vi "BI_VFFT plot 0.5.vi"() -> ()   [LabVIEW 2021]
uses:
  <vilib>/Utility/file.llb/Read Delimited Spreadsheet (DBL).vi
panel:
  out "IV":cluster{dbl[], "Intensity V vs I and B":dbl[]}(graph)
  out "Intensity V vs I and B":dbl[][](graph)
  out "Intensity FFT vs B with fix I":dbl[][](graph)
  out "FFT at fix B and I":cluster{dbl[], "Intensity V vs I and B":dbl[]}(graph)
  out "Intensity FFT vs I with fix B":dbl[][](graph)
  out "FFT at fix I and B":cluster{dbl[], "Intensity V vs I and B":dbl[]}(graph)
  out "I index":i32=30
  out "B index":i32=11
  out "parameter rows":dbl[][](array[numeric])
  out "data rows":dbl[][](array[numeric])
  out "field rows":dbl[][](array[numeric])
  out "Cursor I":dbl=0.29559164733178656
  out "Cursor B":dbl=-0.6575098814229249
  in  "Load":bool
  in  "Stop":bool
  in  "Book number":i32=685
  in  "parent data folder":path=path "C:/Users/gyue/Box/Guang Yue uiuc research box folder/data/Contour plot"
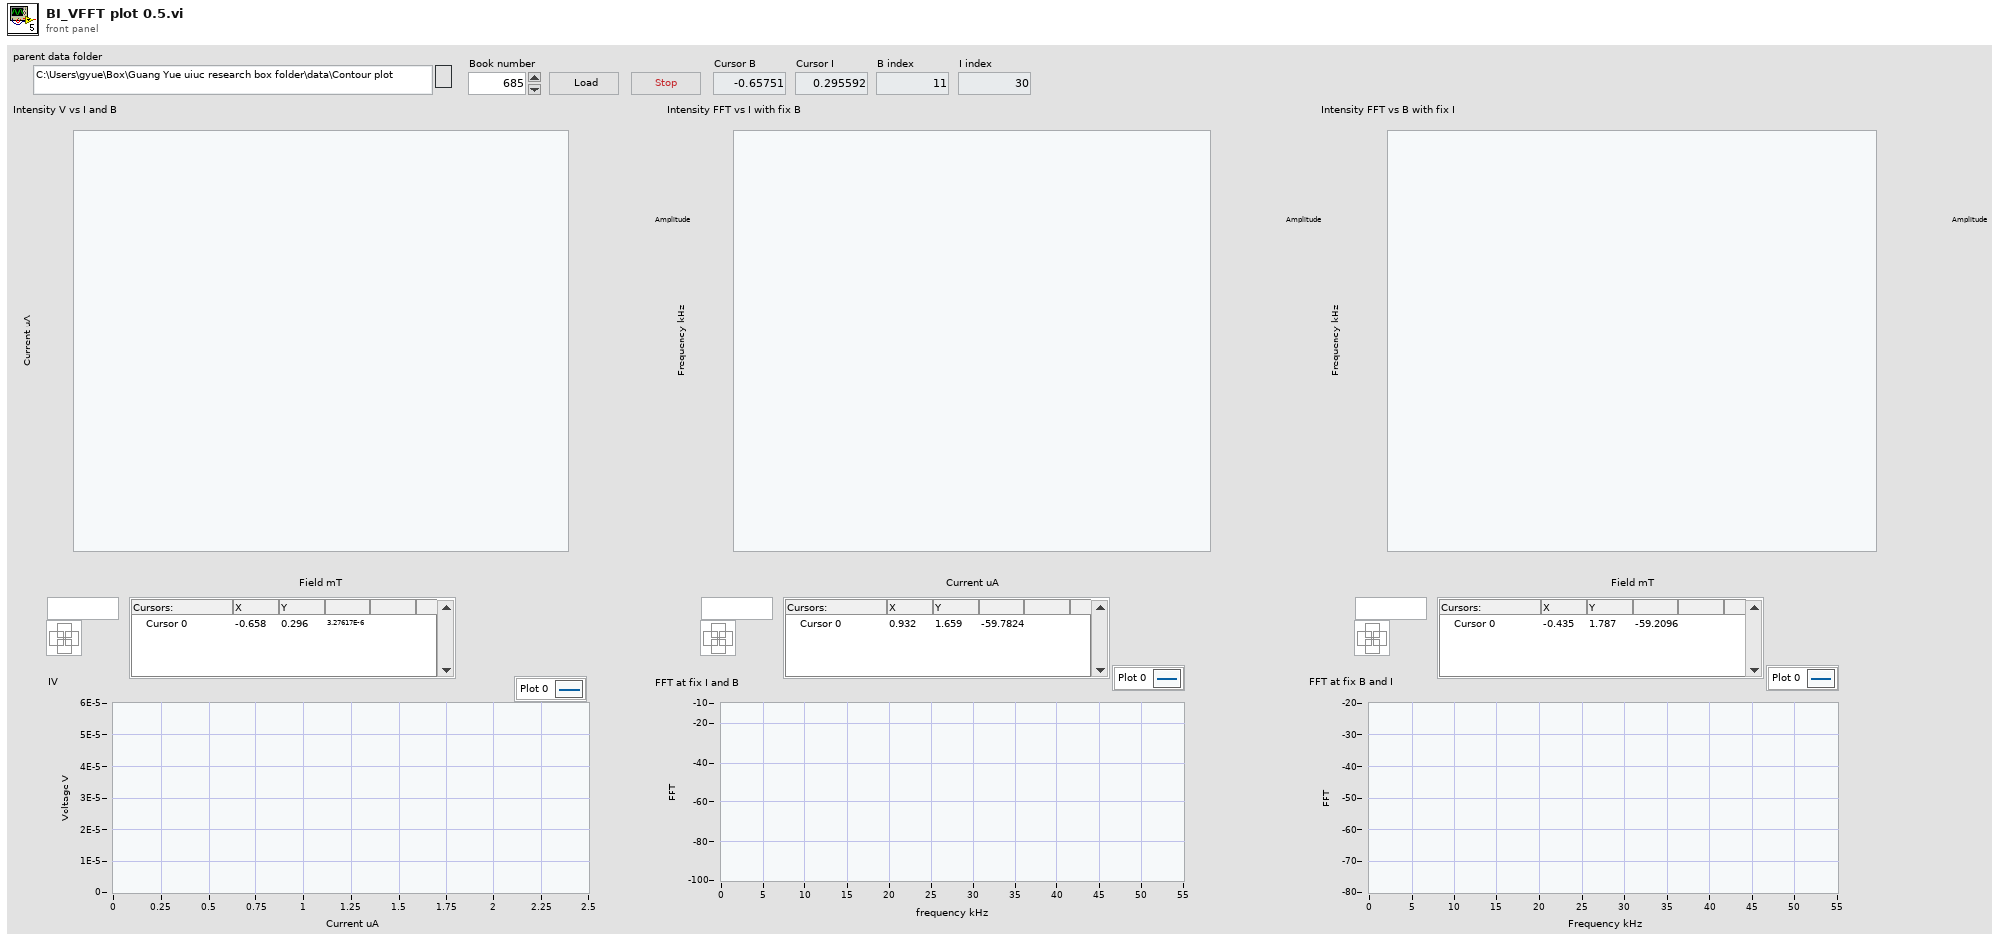
[diagram p1: front panel]
types:
  T1 = cluster{"B offset":dbl, "B multiply":dbl, "I offset":dbl, "I multiply":dbl}
  T2 = cluster{"x offset":dbl, "x multiply":dbl, "y offset":dbl, "y multiply":dbl}
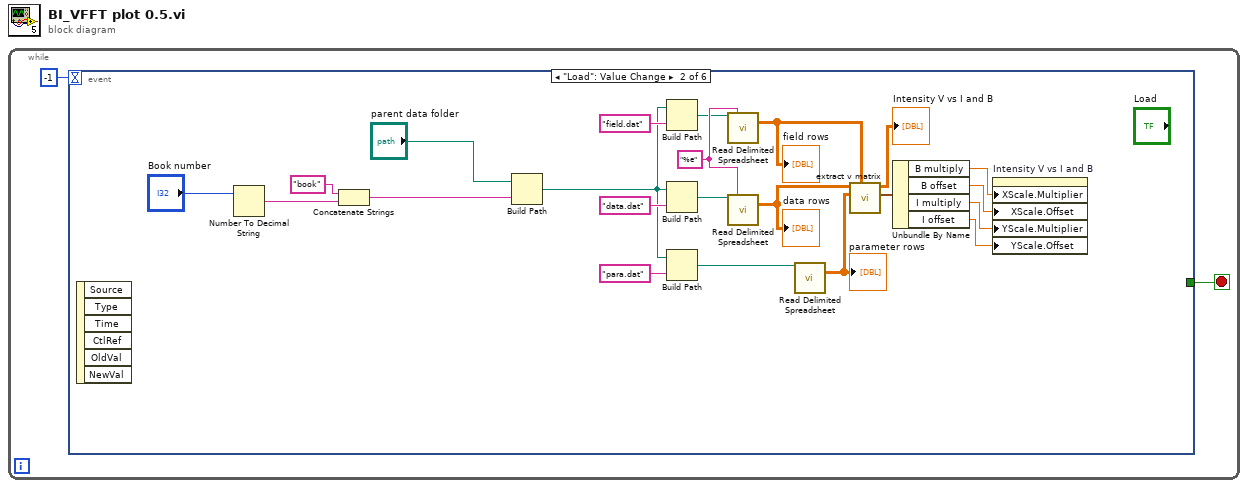
[diagram p0: block diagram]
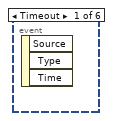
[diagram p2: hidden frame]
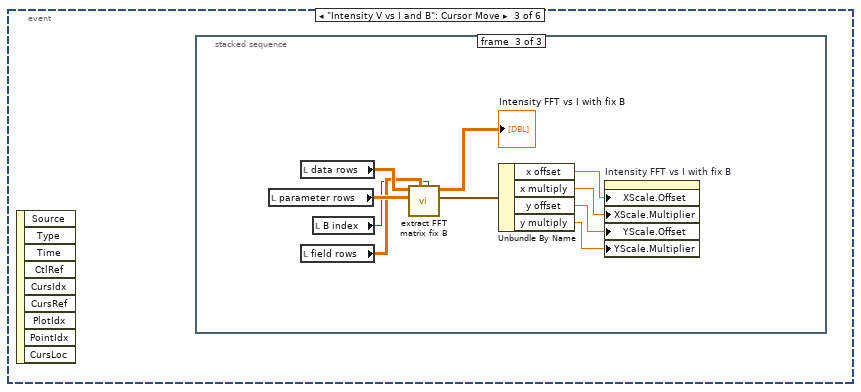
[diagram p3: hidden frame]
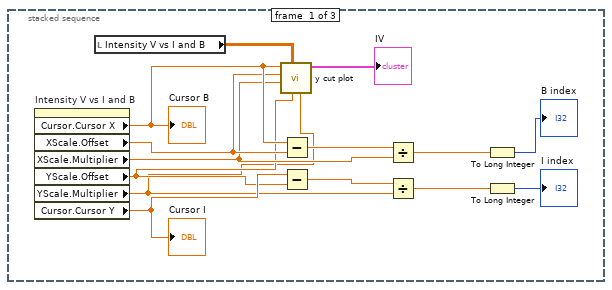
[diagram p4: hidden frame]
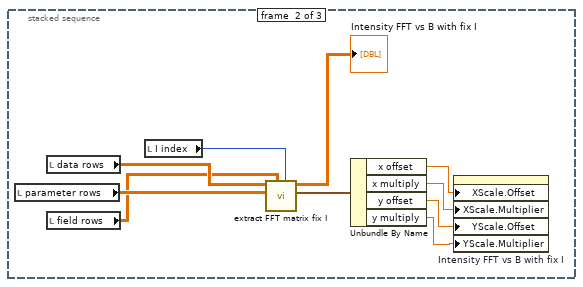
[diagram p5: hidden frame]
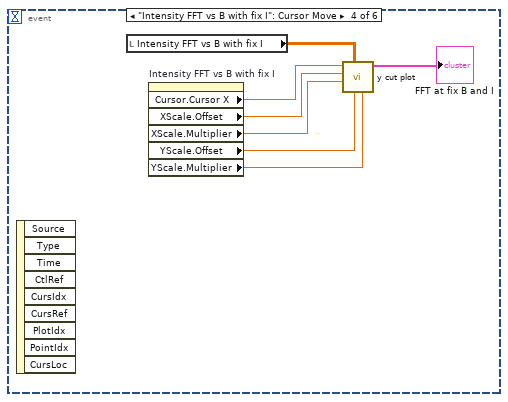
[diagram p6: hidden frame]
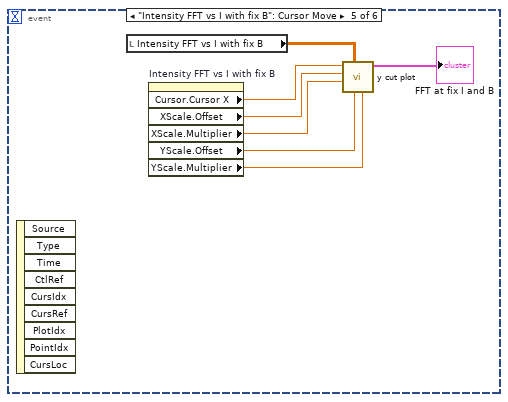
[diagram p7: hidden frame]
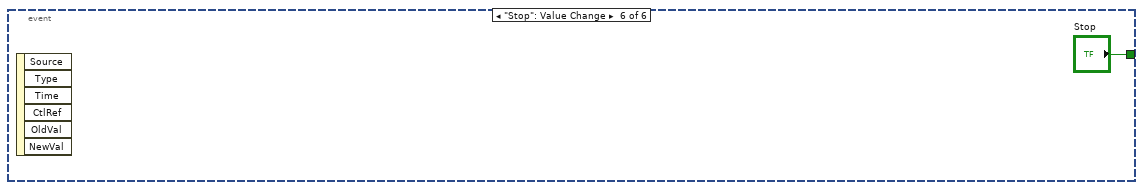
[diagram p8: hidden frame]
diagram:
  n1 = while {
    stop <- w1 stop-if-true
    n2 = event shown="[1] \"Load\": Value Change" {
      selector: _ -> [_ _ _ _ _ _]
      dyn-events: _ -> [_ _ _ _ _ _]
      timeout: -1 -> [_ _ _ _ _ _]
      tunnel: [_ _ _ _ _ "Stop"] -> w1
      event Timeout {
        n3 = event-data() -> ()  [unwired: 1 in, 3 out]
      }
      event "Load": Value Change {
        w15 = "%e" ("format (%.3f)")
        n4 = event-data() -> ()  [unwired: 1 in, 6 out]
        n5 = Number To Decimal String(number="Book number") -> (decimal integer string=w21:string)  [unwired: 1 in]
        n6 = Concatenate Strings("book" ("string"), w21) -> (w20:string)
        n7 = Build Path(base path="parent data folder", name or relative path=w20) -> (appended path=w16:path)
        n8 = Build Path(base path=w16, name or relative path="field.dat") -> (appended path=w13:path)
        n9 = Build Path(base path=w16, name or relative path="data.dat") -> (appended path=w14:path)
        n10 = Build Path(base path=w16, name or relative path="para.dat") -> (appended path=w12:path)
        n11 = call-poly <vilib>:"Read Delimited Spreadsheet.vi"("file path (dialog if empty)"=w13, "format (%.3f)"=w15) -> ("all rows"=w3:dbl[][])  [unwired: 8 in, 5 out]
        "field rows" <- w3
        n12 = call-poly <vilib>:"Read Delimited Spreadsheet.vi"("file path (dialog if empty)"=w14, "format (%.3f)"=w15) -> ("all rows"=w10:dbl[][])  [unwired: 8 in, 5 out]
        "data rows" <- w10
        n13 = call-poly <vilib>:"Read Delimited Spreadsheet.vi"("file path (dialog if empty)"=w12) -> ("all rows"=w11:dbl[][])  [unwired: 9 in, 5 out]
        "parameter rows" <- w11
        n14 = call "extract v matrix.vi"("all field rows"=w3, "parameter"=w11, "all data rows"=w10) -> ("plot parameter"=w8:T1, "V matrix"=→"Intensity V vs I and B":dbl[][])  [unwired: 7 in]
        n15 = Unbundle By Name(w8) -> ("B multiply"=w7:dbl, "B offset"=w6:dbl, "I multiply"=w5:dbl, "I offset"=w4:dbl)
        n16 = property on="Intensity V vs I and B" class="IntGraph (strict)"("XScale.Multiplier"=w7, "XScale.Offset"=w6, "YScale.Multiplier"=w5, "YScale.Offset"=w4) -> ()  [unwired: 2 in, 2 out]
      }
      event "Intensity V vs I and B": Cursor Move {
        n17 = event-data() -> ()  [unwired: 1 in, 9 out]
        n18 = stacked-sequence {
          frame #0 {
            n19 = property on="Intensity V vs I and B" class="IntGraph (strict)"() -> ("Cursor.Cursor X"=w36:dbl, "XScale.Offset"=w35:dbl, "XScale.Multiplier"=w33:dbl, "YScale.Offset"=w27:dbl, "YScale.Multiplier"=w26:dbl, "Cursor.Cursor Y"=w28:dbl)  [unwired: 2 in, 2 out]
            "Cursor B" <- w36
            "Cursor I" <- w28
            n20 = local read "Intensity V vs I and B"() -> (w38:dbl[][])
            n21 = call "y cut plot.vi"("YScale.Multiplier"=w26, "YScale.Offset"=w27, "Intensity V vs I and B"=w38, "XScale.Multiplier"=w33, "XScale.Offset"=w35, "Cursor.Cursor X"=w36) -> ("Cluster"=→"IV":cluster{dbl[], "Intensity V vs I and B":dbl[]})  [unwired: 5 in]
            n22 = Subtract(x=w36, y=w35) -> (x-y=w34:dbl)
            n23 = Subtract(x=w28, y=w27) -> (x-y=w30:dbl)
            n24 = Divide(x=w34, y=w33) -> (x/y=w32:dbl)
            n25 = Divide(x=w30, y=w26) -> (x/y=w29:dbl)
            n26 = To Long Integer(number=w32) -> (32bit integer=→"B index":i32)
            n27 = To Long Integer(number=w29) -> (32bit integer=→"I index":i32)
          }
          frame #1 {
            n28 = local read "parameter rows"() -> (w47:dbl[][])
            n29 = local read "data rows"() -> (w48:dbl[][])
            n30 = local read "field rows"() -> (w46:dbl[][])
            n31 = local read "I index"() -> (w44:i32)
            n32 = call "extract FFT matrix fix I.vi"("I index"=w44, "all field rows"=w46, "parameter"=w47, "all data rows"=w48) -> ("plot parameter"=w45:T2, "FFT matrix"=→"Intensity FFT vs B with fix I":dbl[][])  [unwired: 6 in]
            n33 = Unbundle By Name(w45) -> ("x offset"=w42:dbl, "x multiply"=w41:dbl, "y offset"=w40:dbl, "y multiply"=w39:dbl)
            n34 = property on="Intensity FFT vs B with fix I" class="IntGraph (strict)"("XScale.Offset"=w42, "XScale.Multiplier"=w41, "YScale.Offset"=w40, "YScale.Multiplier"=w39) -> ()  [unwired: 2 in, 2 out]
          }
          frame #2 {
            n35 = local read "parameter rows"() -> (w57:dbl[][])
            n36 = local read "data rows"() -> (w58:dbl[][])
            n37 = local read "field rows"() -> (w56:dbl[][])
            n38 = local read "B index"() -> (w55:i32)
            n39 = call "extract FFT matrix fix B.vi"("B index"=w55, "all field rows"=w56, "parameter"=w57, "all data rows"=w58) -> ("plot parameter"=w53:T2, "FFT matrix"=→"Intensity FFT vs I with fix B":dbl[][])  [unwired: 6 in]
            n40 = Unbundle By Name(w53) -> ("x offset"=w52:dbl, "x multiply"=w51:dbl, "y offset"=w50:dbl, "y multiply"=w49:dbl)
            n41 = property on="Intensity FFT vs I with fix B" class="IntGraph (strict)"("XScale.Offset"=w52, "XScale.Multiplier"=w51, "YScale.Offset"=w50, "YScale.Multiplier"=w49) -> ()  [unwired: 2 in, 2 out]
          }
        }
      }
      event "Intensity FFT vs B with fix I": Cursor Move {
        n42 = event-data() -> ()  [unwired: 1 in, 9 out]
        n43 = local read "Intensity FFT vs B with fix I"() -> (w65:dbl[][])
        n44 = property on="Intensity FFT vs B with fix I" class="IntGraph (strict)"() -> ("Cursor.Cursor X"=w64:dbl, "XScale.Offset"=w63:dbl, "XScale.Multiplier"=w62:dbl, "YScale.Offset"=w60:dbl, "YScale.Multiplier"=w59:dbl)  [unwired: 2 in, 2 out]
        n45 = call "y cut plot.vi"("YScale.Multiplier"=w59, "YScale.Offset"=w60, "Intensity V vs I and B"=w65, "XScale.Multiplier"=w62, "XScale.Offset"=w63, "Cursor.Cursor X"=w64) -> ("Cluster"=→"FFT at fix B and I":cluster{dbl[], "Intensity V vs I and B":dbl[]})  [unwired: 5 in]
      }
      event "Intensity FFT vs I with fix B": Cursor Move {
        n46 = event-data() -> ()  [unwired: 1 in, 9 out]
        n47 = local read "Intensity FFT vs I with fix B"() -> (w72:dbl[][])
        n48 = property on="Intensity FFT vs I with fix B" class="IntGraph (strict)"() -> ("Cursor.Cursor X"=w71:dbl, "XScale.Offset"=w70:dbl, "XScale.Multiplier"=w69:dbl, "YScale.Offset"=w68:dbl, "YScale.Multiplier"=w67:dbl)  [unwired: 2 in, 2 out]
        n49 = call "y cut plot.vi"("YScale.Multiplier"=w67, "YScale.Offset"=w68, "Intensity V vs I and B"=w72, "XScale.Multiplier"=w69, "XScale.Offset"=w70, "Cursor.Cursor X"=w71) -> ("Cluster"=→"FFT at fix I and B":cluster{dbl[], "Intensity V vs I and B":dbl[]})  [unwired: 5 in]
      }
      event "Stop": Value Change {
        n50 = event-data() -> ()  [unwired: 1 in, 6 out]
      }
    }
  }
